vi "FanOnToCloud.vi"() -> ()   [LabVIEW 2020]
uses:
  <vilib>/httpClient/LabVIEWHTTPClient.lvlib
panel:
  in  "FAN ON":bool
  in  "API Key":string
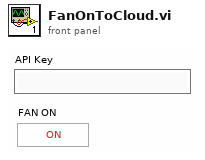
[diagram p1: front panel]
types:
  T1 = typedef "LabVIEWHTTPClient.lvlib/ClientHandle.ctl" = refnum<k1>
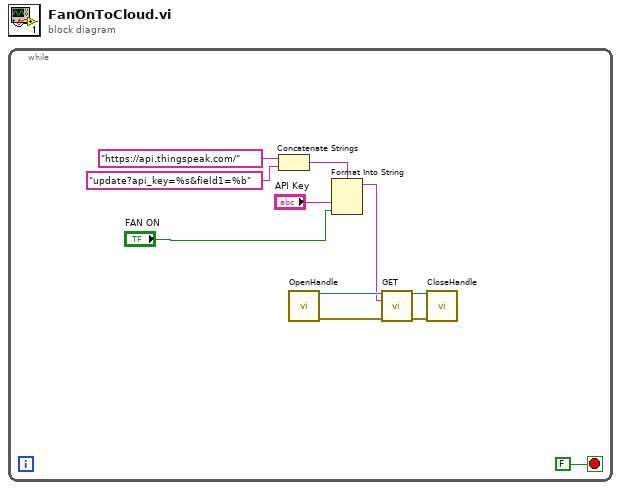
[diagram p0: block diagram]
diagram:
  n1 = while {
    stop <- FALSE stop-if-true
    n2 = Concatenate Strings("https://api.thingspeak.com/" ("string"), "update?api_key=%s&field1=%b" ("string")) -> (w7:string)
    n3 = call <vilib>:"OpenHandle.vi"() -> ("client handle out"=w11:T1, "error out"=w9:errorcluster)  [unwired: 14 in]
    n4 = Format Into String(format string=w7, "API Key", "FAN ON") -> (resulting string=w4:string)  [unwired: 2 in, 1 out]
    n5 = call <vilib>:"GET.vi"("client handle"=w11, "url"=w4, "error in (no error)"=w9) -> ("client handle out"=w10:T1, "error out"=w8:errorcluster)  [unwired: 9 in, 2 out]
    n6 = call <vilib>:"CloseHandle.vi"("client handle"=w10, "error in (no error)"=w8) -> ()  [unwired: 13 in, 1 out]
  }
